vi "GetArrayElement.vi"(6 "error in":errorcluster, 9 "Array in":refnum<class "Array.lvclass">) -> (0 "error out":errorcluster, 3 "Array out":refnum<class "Array.lvclass">, 4 "Array Element":i32)   [LabVIEW 2014, in "Raspberry Pi Compatible Compiler for LabVIEW.lvlib" / "Array.lvclass"]
uses:
  Array.lvclass
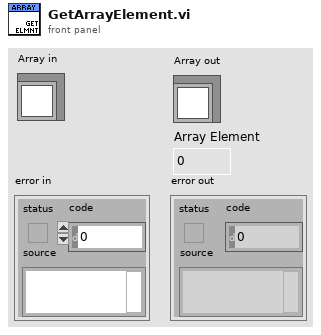
[diagram p1: front panel]
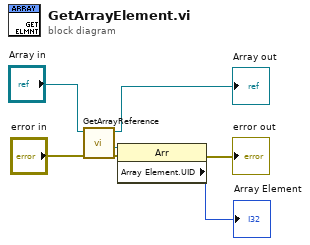
[diagram p0: block diagram]
diagram:
  n1 = call "GetArrayReference.vi"("error in"="error in", "Array in"="Array in") -> ("error out"=w3:errorcluster, "array reference"=w4:refnum<vi>, "Array out"=→"Array out":refnum<class "Array.lvclass">)  [unwired: 7 in]
  n2 = property class="Arr"(reference=w4, error in=w3) -> (error out=→"error out":errorcluster, "Array Element.UID"=→"Array Element":i32)  [unwired: 1 out]
